vi "tasterino.vi"() -> ()   [LabVIEW 2017]
panel:
  in  "Boolean 4":bool
  in  "Boolean 3":bool
  in  "Boolean 2":bool
  in  "Boolean":bool
  out "String":string
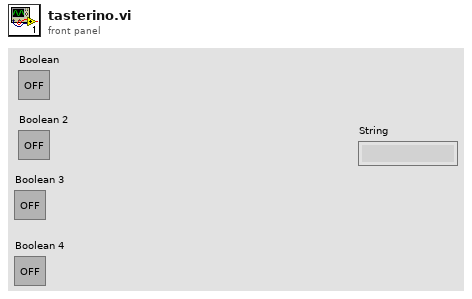
[diagram p1: front panel]
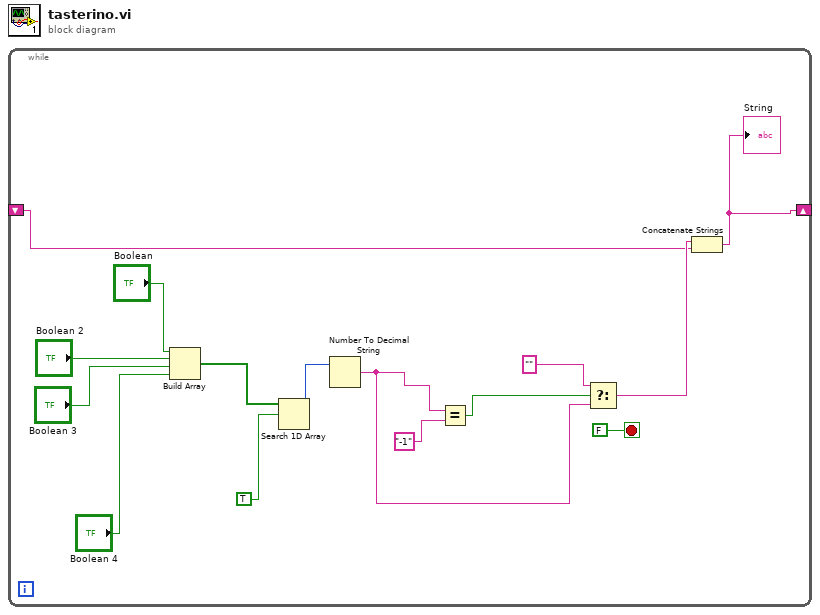
[diagram p0: block diagram]
diagram:
  n1 = while {
    shift-right: [w3] -> _
    shift-left: _ -> [w1]
    stop <- FALSE stop-if-true
    n2 = Build Array("Boolean", "Boolean 2", "Boolean 3", "Boolean 4") -> (w14:bool[])
    n3 = Search 1D Array(1D array=w14, element=TRUE) -> (index of element=w7:i32)  [unwired: 1 in]
    n4 = Number To Decimal String(number=w7) -> (decimal integer string=w9:string)  [unwired: 1 in]
    n5 = Equal?(x=w9, y="-1") -> (x = y?=w8:bool)
    n6 = Select(t="" ("f"), s=w8, f=w9) -> (s? t:f=w2:string)
    n7 = Concatenate Strings(w2, w1) -> (w3:string)
    "String" <- w3
  }
